vi "IDE.vi"() -> ()   [LabVIEW 2020]
uses:
  Subs/ColorText/Code.xctl
  Subs/Console XCtrl/Console_Xctrl.xctl
  Subs/Server XCtrl/Server.xctl
panel:
  in  "New":bool
  in  "Tree":string(tree)
  in  "Clean":bool
  in  "PC Save":bool
  in  "Base path":path
  in  "Files":bool
  in  "Server":bool
  in  "Help":bool
  in  "Server":path(xcontrol)=path "/Users/CarterWS/Desktop/Senior Spring/CEEO/Summer2020/LabVIEWCode/Servers/Peter.vi"
  out "REPL":string(xcontrol)
  in  "Clear":bool
  in  "Save":bool
  in  "Stop":bool
  in  "Run":bool=TRUE
  in  "Name":string="test.py"
  in  "Code":string(xcontrol)="#!/usr/bin/env pybricks-micropython\n\nfrom pybricks import ev3brick as brick\nfrom pybricks.ev3devices import (Motor, TouchSensor, \n    ColorSensor,InfraredSensor, UltrasonicSensor, GyroSensor)\nfrom pybricks.parameters import (Port, Stop, Direction, Button, Color,\n    SoundFile, ImageFile, Align)\nfrom pybricks.tools import print, wait, StopWatch\nfrom pybricks.robotics import DriveBase\nimport time\n"
  # "¨Processor"
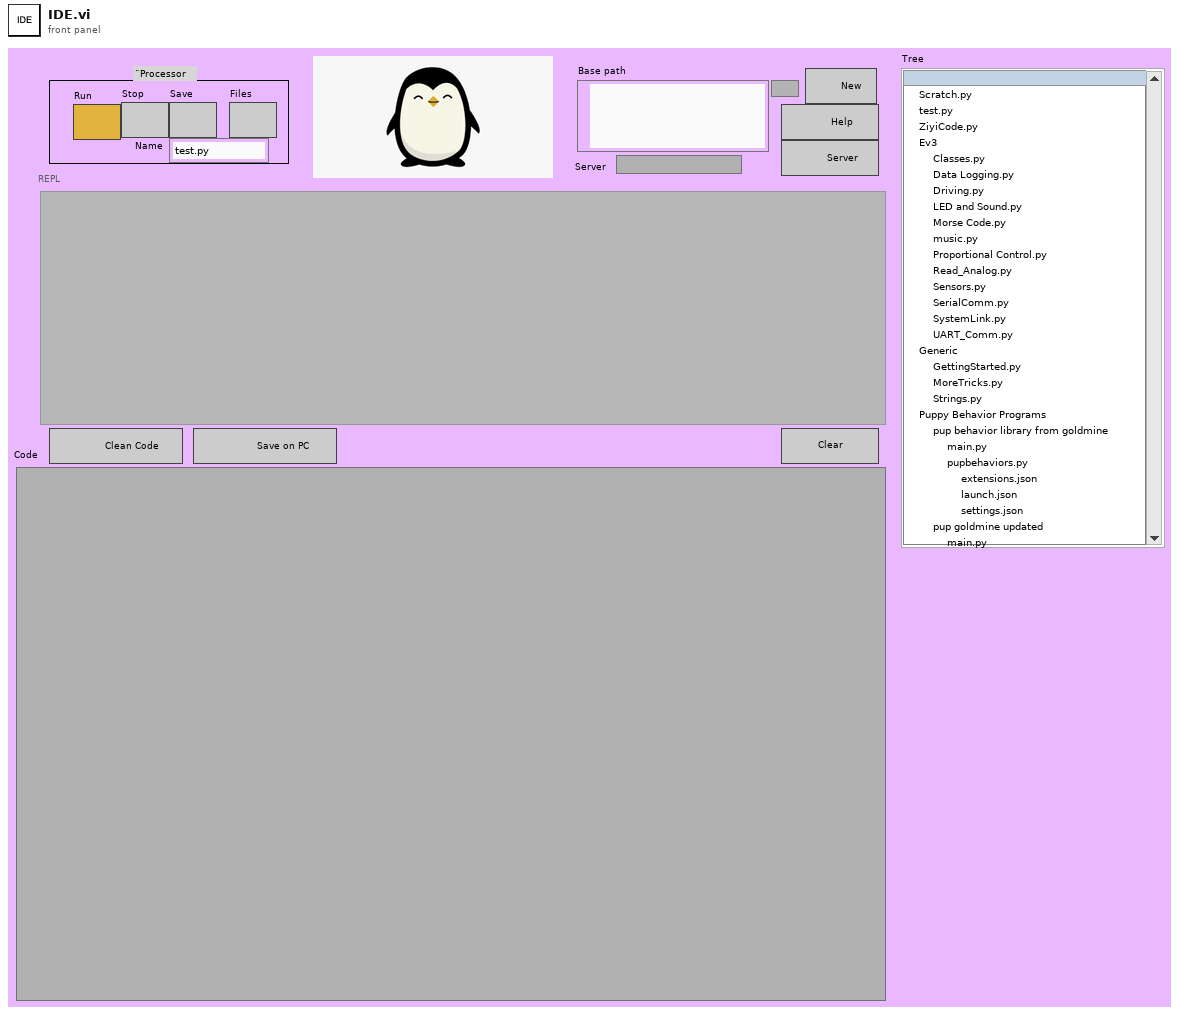
[diagram p1: front panel]
types:
  T1 = cluster{"Quote":u32, "Comment":u32, "Python":u32, "Text":u32, "Triple Quote":u32, "function":u32, "Line numbers":u32, "REPL Err":u32, "REPL Text":u32, "Text Bkgd":u32, "REPL Bkgd":u32}
  T2 = enum8{"Enabled", "Disabled", "Disabled and Grayed Out"}
  T3 = typedef "eventvkey.ctl" = enum16{"ASCII", "Enter", "Return", "Shift", "Ctrl", "Alt", "Cmd", "Opt", "Caps", "NumLock", "Clear", "Break", "Up", "Down", "Left", "Right", "Insert", "Delete", "Home", "End", "PageUp", "PageDown", "Escape", "Help", "Pause", "ScrollLock", "F1", "F2", "F3", "F4", "F5", "F6", "F7", "F8", "F9", "F10", "F11", "F12", "F13", "F14", "F15", "F16", "F17", "F18", "F19", "F20", "F21", "F22", "F23", "F24", "Play", "VolumeUp", "VolumeDown", "Mute", "Two Byte Char"}
  T4 = cluster{"Shift":bool, "Ctrl":bool, "Alt":bool, "Cmd":bool, "Opt":bool}
  T5 = cluster{"Char":i16, "VKey":T3, "PlatMods":cluster{"Shift":bool, "Ctrl":bool, "Alt":bool, "Cmd":bool, "Opt":bool}}
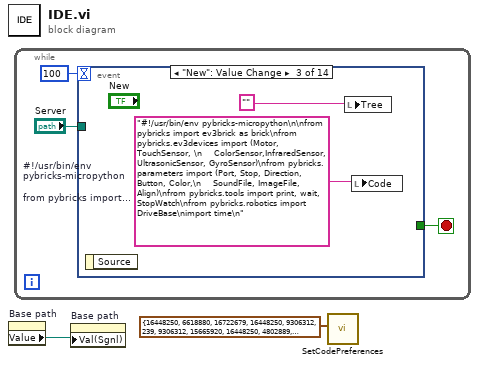
[diagram p0: block diagram]
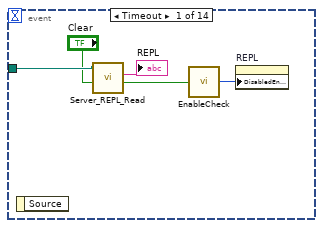
[diagram p2: hidden frame]
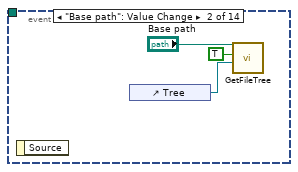
[diagram p3: hidden frame]
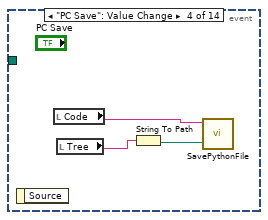
[diagram p4: hidden frame]
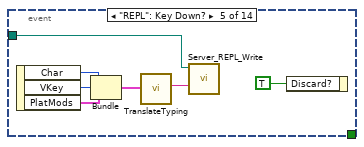
[diagram p5: hidden frame]
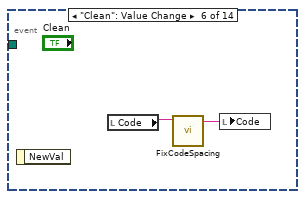
[diagram p6: hidden frame]
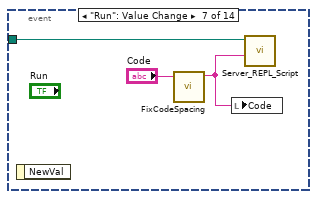
[diagram p7: hidden frame]
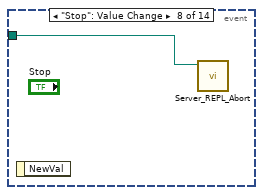
[diagram p8: hidden frame]
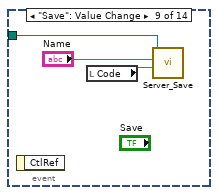
[diagram p9: hidden frame]
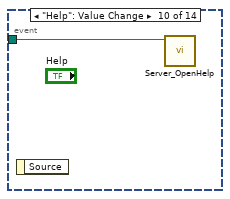
[diagram p10: hidden frame]
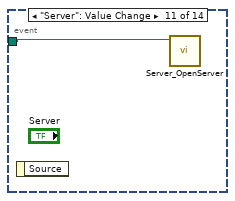
[diagram p11: hidden frame]
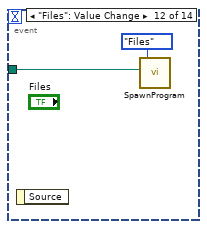
[diagram p12: hidden frame]
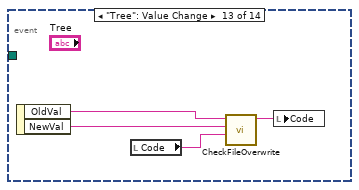
[diagram p13: hidden frame]
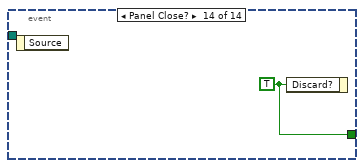
[diagram p14: hidden frame]
diagram:
  n1 = property on="Base path" class="Path"() -> ("Value"=w1:path)  [unwired: 2 in, 2 out]
  n2 = while {
    stop <- w4 stop-if-true
    n3 = event shown="[2] \"New\": Value Change" {
      selector: _ -> [_ _ _ _ _ _ _ _ _ _ _ _ _ _]
      dyn-events: _ -> [_ _ _ _ _ _ _ _ _ _ _ _ _ _]
      timeout: 100 -> [_ _ _ _ _ _ _ _ _ _ _ _ _ _]
      tunnel: [_ _ _ _ _ _ _ _ _ _ _ _ _ w43] -> w4
      tunnel: "Server" -> [w8 _ _ _ w19 _ w29 w31 w32 w35 w36 w37 _ _]
      event Timeout {
        n4 = event-data() -> ()  [unwired: 1 in, 1 out]
        n5 = call "Server_REPL_Read.vi"("Clear"="Clear", "Server"=w8) -> ("Running?"=w9:bool, "REPL"=→"REPL":string)  [unwired: 7 in, 1 out]
        n6 = call "EnableCheck.vi"("Enable?"=w9) -> ("Enum"=w10:T2)
        n7 = property on="REPL" class="Console_Xctrl (strict)"("DisabledEnum"=w10) -> ()  [unwired: 2 in, 2 out]
      }
      event "Base path": Value Change {
        n8 = event-data() -> ()  [unwired: 1 in, 1 out]
        n9 = control-ref of="Tree"() -> (w12:refnum<vi>)
        n10 = call "GetFileTree.vi"("Tree"=w12, "Open?"=TRUE, "Base Path"="Base path") -> ()  [unwired: 9 in]
      }
      event "New": Value Change {
        w14 = "#!/usr/bin/env pybricks-micropython\n\nfrom pybricks import ev3brick as brick\nfrom pybricks.ev3devices import (Motor, TouchSensor, \n    ColorSensor,InfraredSensor, UltrasonicSensor, GyroSensor)\nfrom pybricks.parameters import (Port, Stop, Direction, Button, Color,\n    SoundFile, ImageFile, Align)\nfrom pybricks.tools import print, wait, StopWatch\nfrom pybricks.robotics import DriveBase\nimport time\n"  # #!/usr/bin/env pybricks-micropython  from pybricks import ev3brick as brick from pybricks.ev3devices import (Motor, TouchSensor,      ColorSensor,InfraredSensor, UltrasonicSensor, GyroSensor) from pybricks.parameters import (Port, Stop, Direction, Button, Color,     SoundFile, ImageFile, Align) from pybricks.tools import print, wait, StopWatch from pybricks.robotics import DriveBase import time
        n11 = event-data() -> ()  [unwired: 1 in, 1 out]
        n12 = local write "Tree"("") -> ()
        n13 = local write "Code"(w14) -> ()
      }
      event "PC Save": Value Change {
        n14 = event-data() -> ()  [unwired: 1 in, 1 out]
        n15 = local read "Code"() -> (w17:string)
        n16 = local read "Tree"() -> (w18:string)
        n17 = String To Path(string=w18) -> (path=w16:path)
        n18 = call "SavePythonFile.vi"("path"=w16, "Code"=w17) -> ()  [unwired: 10 in]
      }
      event "REPL": Key Down? {
        n19 = event-data() -> ("Char"=w24:i16, "VKey"=w23:T3, "PlatMods"=w21:T4)  [unwired: 1 in]
        n20 = Bundle("Char"=w24, "VKey"=w23, "PlatMods"=w21) -> (w25:T5)  [unwired: 1 in]
        n21 = call "TranslateTyping.vi"("Cluster"=w25) -> ("key"=w20:string)  [unwired: 10 in]
        n22 = call "Server_REPL_Write.vi"("Code"=w20, "Server"=w19) -> ()  [unwired: 9 in, 1 out]
        n23 = event-data("Discard?"=TRUE) -> ()  [unwired: 1 in, 1 out]
      }
      event "Clean": Value Change {
        n24 = event-data() -> ()  [unwired: 1 in, 1 out]
        n25 = local read "Code"() -> (w26:string)
        n26 = call "FixCodeSpacing.vi"("Code"=w26) -> ("Cleaned"=w27:string)  [unwired: 10 in]
        n27 = local write "Code"(w27) -> ()
      }
      event "Run": Value Change {
        n28 = event-data() -> ()  [unwired: 1 in, 1 out]
        n29 = call "FixCodeSpacing.vi"("Code"="Code") -> ("Cleaned"=w28:string)  [unwired: 10 in]
        n30 = local write "Code"(w28) -> ()
        n31 = call "Server_REPL_Script.vi"("Code"=w28, "Server"=w29) -> ()  [unwired: 9 in, 1 out]
      }
      event "Stop": Value Change {
        n32 = event-data() -> ()  [unwired: 1 in, 1 out]
        n33 = call "Server_REPL_Abort.vi"("Server"=w31) -> ()  [unwired: 10 in, 1 out]
      }
      event "Save": Value Change {
        n34 = event-data() -> ()  [unwired: 1 in, 1 out]
        n35 = local read "Code"() -> (w34:string)
        n36 = call "Server_Save.vi"("Code"=w34, "Name"="Name", "Server"=w32) -> ()  [unwired: 8 in, 1 out]
      }
      event "Help": Value Change {
        n37 = event-data() -> ()  [unwired: 1 in, 1 out]
        n38 = call "Server_OpenHelp.vi"("Server"=w35) -> ()  [unwired: 10 in, 1 out]
      }
      event "Server": Value Change {
        n39 = event-data() -> ()  [unwired: 1 in, 1 out]
        n40 = call "Server_OpenServer.vi"("Server"=w36) -> ()  [unwired: 10 in, 1 out]
      }
      event "Files": Value Change {
        n41 = event-data() -> ()  [unwired: 1 in, 1 out]
        n42 = call "SpawnProgram.vi"("Server"=w37, "Dialog"=enum16{"Help", "Files"}."Files") -> ()  [unwired: 10 in]
      }
      event "Tree": Value Change {
        n43 = event-data() -> ("OldVal"=w40:string, "NewVal"=w39:string)  [unwired: 1 in]
        n44 = local read "Code"() -> (w41:string)
        n45 = call "CheckFileOverwrite.vi"("Current Code"=w41, "New Value"=w39, "Old Value"=w40) -> ("Code out"=w42:string)  [unwired: 8 in]
        n46 = local write "Code"(w42) -> ()
      }
      event Panel Close? {
        w43 = TRUE ("Discard?")
        n47 = event-data() -> ()  [unwired: 1 in, 1 out]
        n48 = event-data("Discard?"=w43) -> ()  [unwired: 1 in, 1 out]
      }
    }
  }
  n49 = property on="Base path" class="Path"("Val(Sgnl)"=w1) -> ()  [unwired: 2 in, 2 out]
  n50 = call "SetCodePreferences.vi"("Color choices"=T1 {"Quote"=16448250, "Comment"=6618880, "Python"=16722679, "Text"=16448250, "Triple Quote"=9306312, "function"=239, "Line numbers"=9306312, "REPL Err"=15665920, "REPL Text"=16448250, "Text Bkgd"=4802889, "REPL Bkgd"=4802889}) -> ()  [unwired: 11 in]
